vi "DR_Event.vi"(4 "DR_DataQ":refnum<queue>, 5 "Event Data":cluster{"record":variant}, 6 "Control Ref":refnum<k7>, 7 "Event Common Data":T1) -> ()   [LabVIEW 2015]
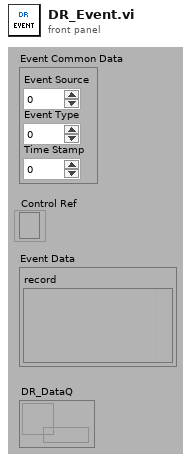
[diagram p1: front panel]
types:
  T1 = cluster{"Event Source":i32, "Event Type":u32, "Time Stamp":u32}
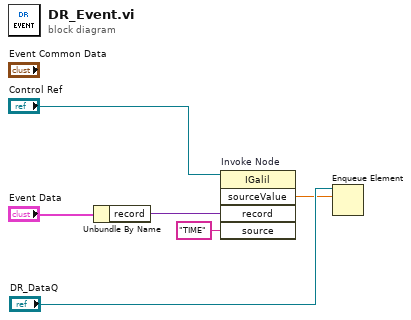
[diagram p0: block diagram]
diagram:
  n1 = Unbundle By Name("Event Data") -> ("record"=w4:variant)
  n2 = invoke on="Invoke Node" class="IGalil" method="sourceValue"(reference="Control Ref", "record"=w4, "source"="TIME") -> ("sourceValue"=w1:dbl)  [unwired: 2 in, 4 out]
  n3 = Enqueue Element(queue="DR_DataQ", element=w1) -> ()  [unwired: 2 in, 3 out]
